vi "Count.vi"(4 "error in":errorcluster, 7 "Counter task":refnum<k21>) -> (0 "error out":errorcluster, 2 "Counts":dbl, 3 "Counter task out":refnum<k21>)   [LabVIEW 2010]
uses:
  <vilib>/DAQmx/read.llb/DAQmx Read (Counter DBL 1Chan 1Samp).vi
  <vilib>/daqmx/miscellaneous.llb/DAQmx Fill In Error Info.vi
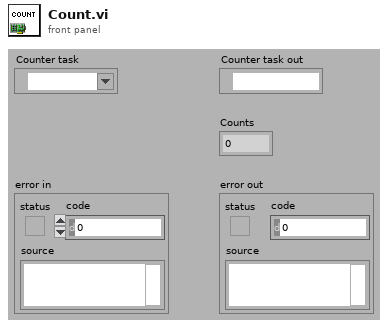
[diagram p1: front panel]
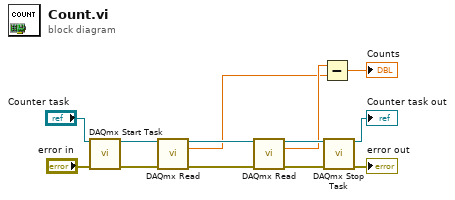
[diagram p0: block diagram]
diagram:
  n1 = call <vilib>:"DAQmx Start Task.vi"("task/channels in"="Counter task", "error in"="error in") -> ("task out"=w7:refnum<k21>, "error out"=w8:errorcluster)  [unwired: 12 out]
  n2 = call-poly <vilib>:"DAQmx Read.vi"("task/channels in"=w7, "error in"=w8) -> ("task out"=w6:refnum<k21>, "data"=w1:dbl, "error out"=w4:errorcluster)  [unwired: 11 out]
  n3 = call-poly <vilib>:"DAQmx Read.vi"("task/channels in"=w6, "error in"=w4) -> ("task out"=w5:refnum<k21>, "data"=w2:dbl, "error out"=w3:errorcluster)  [unwired: 11 out]
  n4 = Subtract(x=w2, y=w1) -> (x-y=→"Counts":dbl)
  n5 = call <vilib>:"DAQmx Stop Task.vi"("task/channels in"=w5, "error in"=w3) -> ("task out"=→"Counter task out":refnum<k21>, "error out"=→"error out":errorcluster)  [unwired: 12 out]
